vi "getBitAsNumeric.vi"(10 "n":i32=-1, 11 "input":u8 format="%08b") -> (3 "bit":u8 format="%01b")   [LabVIEW 2013, in "bitwiseOps.lvlib"]
uses:
  bitwiseOps.lvlib
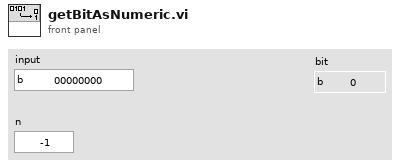
[diagram p1: front panel]
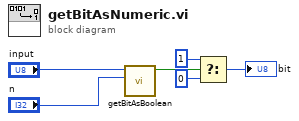
[diagram p0: block diagram]
diagram:
  n1 = call "getBitAsBoolean.vi"("n"="n", "input"="input") -> ("bit"=w1:bool)  [unwired: 9 in]
  n2 = Select(t=u8 1 ("bit"), s=w1, f=u8 0 ("bit")) -> (s? t:f=→"bit":u8)
